vi "MV turn on.vi"(8 "error in (no error)":errorcluster, 11 "VISA resource name":refnum<visa-resource-name>) -> (0 "error out":errorcluster, 3 "VISA resource name out":refnum<visa-resource-name>)   [LabVIEW 2017, in "Millennia V.lvclass"]
doc: "Once the Millennia V is warmed up, use this to turn it on."
uses:
  Millennia V.lvclass
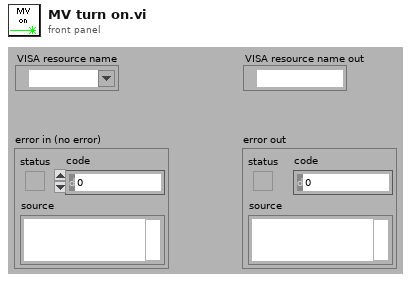
[diagram p1: front panel]
types:
  T1 = enum16{"read only", "write only", "write + read"}
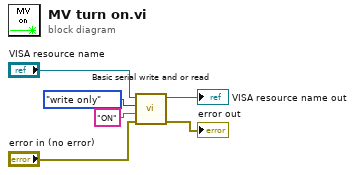
[diagram p0: block diagram]
diagram:
  n1 = call "Basic serial write and or read.vi"("error in (no error)"="error in (no error)", "write string"="ON", "action"=T1."write only", "VISA resource name"="VISA resource name") -> ("error out"=→"error out":errorcluster, "VISA resource name out"=→"VISA resource name out":refnum<visa-resource-name>)  [unwired: 4 in, 2 out]
